vi "ThermalMap.vi"() -> ()   [LabVIEW 2018]
uses:
  <vilib>/Utility/file.llb/Write Delimited Spreadsheet (I64).vi
panel:
  in  "Tab Control":enum32{"File", "Page 2"}(tab)
  in  "Filename":string="Run 0_image"
  out "file path":path=path "M:/Oceanoptics/TDMS test/Spectrometer.csv"
  out "output cluster":cluster{"Image Pixels (U8)":u8[][]}
  in  "Stop":bool
  out "Image Out":T1(plugin-control)
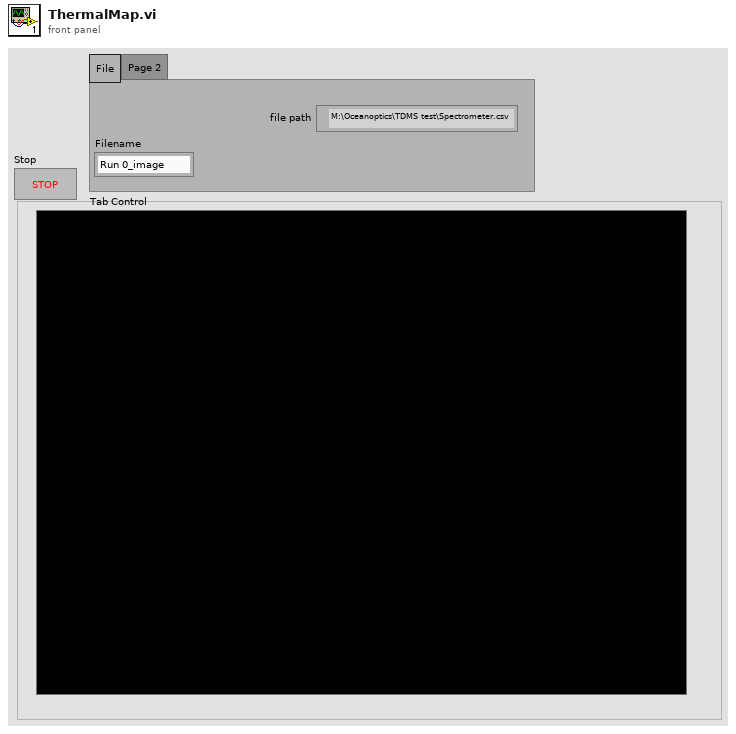
[diagram p1: front panel]
types:
  T1 = typedef "IMAQ Image.ctl" = refnum<image>
  T2 = enum16{"open", "replace", "create", "open or create", "replace or create", "replace or create with confirmation"}
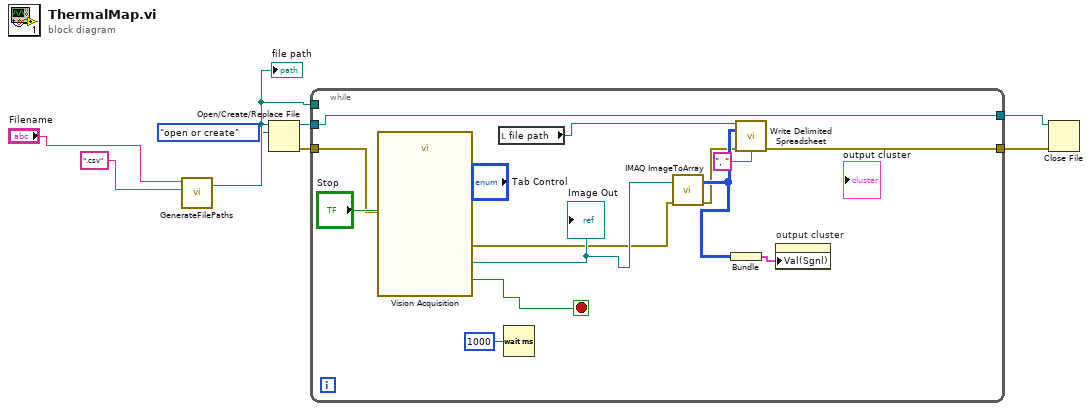
[diagram p0: block diagram]
diagram:
  n1 = call "GenerateFilePaths.vi"("Extension (.tdms)"=".csv", "Device Name"="Filename") -> ("Path"=w2:path)  [unwired: 3 in]
  "file path" <- w2
  n2 = Open/Create/Replace File(file path (use dialog)=w2, operation (0:open)=T2."open or create") -> (refnum out=w8:refnum<file>, error out=w6:errorcluster)  [unwired: 4 in, 1 out]
  n3 = while {
    tunnel: w2 -> [_]
    tunnel: w8 -> [w14]
    tunnel: [w14] -> w7
    tunnel: w6 -> [w13]
    tunnel: [w10] -> w5
    stop <- w21 stop-if-true
    n4 = call "Vision Acquisition"("Stop (F)"="Stop", "error in"=w13) -> ("Image Out"=w19:T1, "Stopped"=w21:bool, "error out"=w12:errorcluster)  [unwired: 23 in]
    "Image Out" <- w19
    n5 = local read "file path"() -> (w16:path)
    n6 = Wait (ms)(milliseconds to wait=u32 1000) -> ()  [unwired: 1 out]
    n7 = call "IMAQ ImageToArray"("error in (no error)"=w12, "Image"=w19) -> ("error out"=w11:errorcluster, "Image Pixels (U8)"=w17:u8[][])  [unwired: 2 in, 3 out]
    n8 = Bundle("Image Pixels (U8)"=w17) -> (w18:cluster{"Image Pixels (U8)":u8[][]})  [unwired: 1 in]
    n9 = call-poly <vilib>:"Write Delimited Spreadsheet.vi"("file path (dialog if empty)"=w16, "2D data"=w17, "error in (no error)"=w11, "delimiter (\\t)"=", " ("delimiter (\\t)")) -> ("error out"=w10:errorcluster)  [unwired: 10 in, 1 out]
    n10 = property on="output cluster" class="Clust (strict)"("Val(Sgnl)"=w18) -> ()  [unwired: 2 in, 2 out]
  }
  n11 = Close File(refnum=w7, error in=w5) -> ()  [unwired: 2 out]
